vi "init joystick.vi"() -> (0 "device ID":refnum<k1>, 1 "Joystick found":bool)   [LabVIEW 2012]
uses:
  <vilib>/Utility/inputDevices.llb/joystickAcquire.vi
  <vilib>/Utility/inputDevices.llb/closeJoystick.vi
panel:
  out "joystick info":T1(array[cluster])
  out "Array":T2(array[cluster])
  out "appended array":i32[](array[numeric])
  out "button info":T3
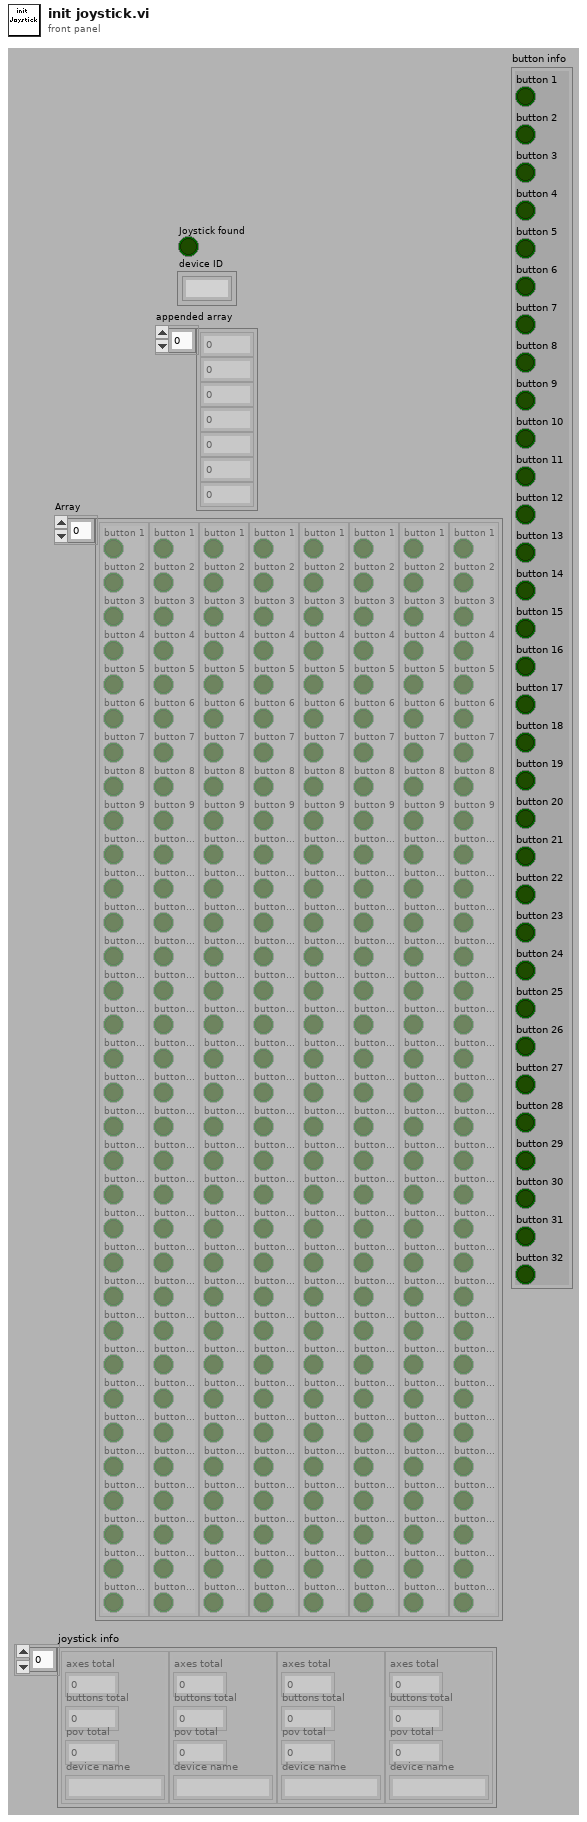
[diagram p1: front panel]
types:
  T1 = cluster{"axes total":u32, "buttons total":u32, "pov total":u32, "device name":string}[]
  T2 = cluster{"button 1":bool, "button 2":bool, "button 3":bool, "button 4":bool, "button 5":bool, "button 6":bool, "button 7":bool, "button 8":bool, "button 9":bool, "button 10":bool, "button 11":bool, "button 12":bool, "button 13":bool, "button 14":bool, "button 15":bool, "button 16":bool, "button 17":bool, "button 18":bool, "button 19":bool, "button 20":bool, "button 21":bool, "button 22":bool, "button 23":bool, "button 24":bool, "button 25":bool, "button 26":bool, "button 27":bool, "button 28":bool, "button 29":bool, "button 30":bool, "button 31":bool, "button 32":bool}[]
  T3 = cluster{"button 1":bool, "button 2":bool, "button 3":bool, "button 4":bool, "button 5":bool, "button 6":bool, "button 7":bool, "button 8":bool, "button 9":bool, "button 10":bool, "button 11":bool, "button 12":bool, "button 13":bool, "button 14":bool, "button 15":bool, "button 16":bool, "button 17":bool, "button 18":bool, "button 19":bool, "button 20":bool, "button 21":bool, "button 22":bool, "button 23":bool, "button 24":bool, "button 25":bool, "button 26":bool, "button 27":bool, "button 28":bool, "button 29":bool, "button 30":bool, "button 31":bool, "button 32":bool}
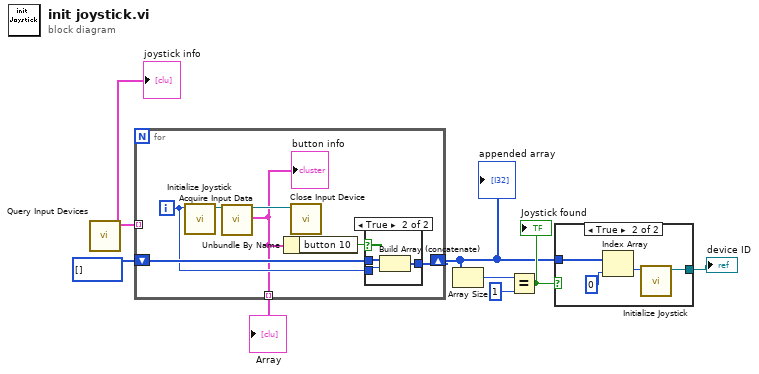
[diagram p0: block diagram]
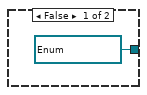
[diagram p2: hidden frame]
diagram:
  n1 = call <vilib>:"Query Input Devices.vi"() -> ("joystick info"=w2:T1)  [unwired: 1 in, 10 out]
  "joystick info" <- w2
  n2 = for {
    shift-right: [w12] -> w4
    shift-left: i32[] [] ("appended array") -> [w13]
    tunnel: w2 -> [_] mode=indexing
    tunnel: [w9] -> w1 mode=indexing
    i -> [w11]
    n3 = call <vilib>:"Initialize Joystick.vi"("device index"=w11) -> ("device ID"=w15:refnum<k1>)  [unwired: 1 in, 9 out]
    n4 = call-poly <vilib>:"Acquire Input Data.vi"("device ID"=w15) -> ("device ID"=w14:refnum<k1>, "button info"=w9:T3)  [unwired: 1 in, 16 out]
    "button info" <- w9
    n5 = Unbundle By Name(w9) -> ("button 10"=w10:bool)
    n6 = call-poly <vilib>:"Close Input Device.vi"("device ID"=w14) -> ()  [unwired: 1 in, 9 out]
    n7 = case shown="True" w10 {
      tunnel: w13 -> [w16 w17]
      tunnel: [w16 w18] -> w12
      tunnel: w11 -> [_ w19]
      frame False {
      }
      frame True {
        n8 = Build Array (concatenate)(w17, w19) -> (w18:i32[])
      }
    }
  }
  "appended array" <- w4
  "Array" <- w1
  n9 = Array Size(array=w4) -> (size(s)=w6:i32)
  n10 = Equal?(x=w6, y=1) -> (x = y?=w5:bool)
  "Joystick found" <- w5
  n11 = case shown="True" w5 {
    tunnel: w4 -> [_ w24]
    tunnel: [w20 w21] -> w3
    frame False {
      w20 = refnum<k1> refnum items=["JOYSTICK"] ("device ID")
    }
    frame True {
      n12 = Index Array(array=w24, index=0) -> (element=w22:i32)
      n13 = call <vilib>:"Initialize Joystick.vi"("device index"=w22) -> ("device ID"=w21:refnum<k1>)  [unwired: 1 in, 9 out]
    }
  }
  "device ID" <- w3
